vi "Extended Power Spectra 2D.vi"(8 "Error In":errorcluster, 9 "Waveforms In":waveform(dbl)[](array[waveform])) -> (0 "Error Out":errorcluster, 1 "Power Spectra":cluster{"f0":dbl, "df":dbl, "Magnitude":dbl[]}[](array[cluster]), 2 "Power Spectra 2":cluster{"f0":dbl, "df":dbl, "Magnitude":dbl[]}, 3 "Power Spectra 1":cluster{"f0":dbl, "df":dbl, "Magnitude":dbl[]})   [LabVIEW 2017]
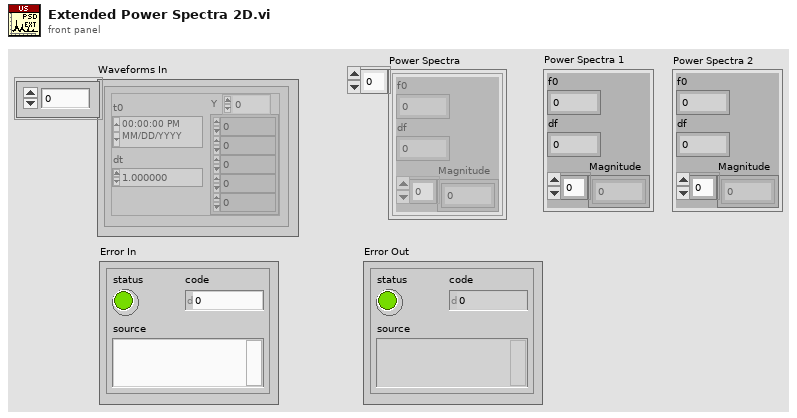
[diagram p1: front panel]
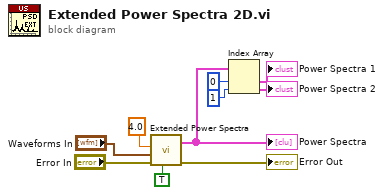
[diagram p0: block diagram]
diagram:
  n1 = call "Extended Power Spectra.vi"("Normalize?"=TRUE, "Error In"="Error In", "Waveforms In"="Waveforms In", "Upsampling pow. of 2"=4.0) -> ("Error Out"=→"Error Out":errorcluster, "Power Spectra"=w7:cluster{"f0":dbl, "df":dbl, "Magnitude":dbl[]}[])  [unwired: 6 in]
  "Power Spectra" <- w7
  n2 = Index Array(array=w7, index #1=0 ("disabled index (col)"), index #2=1 ("index (col)")) -> (element #1=→"Power Spectra 1":cluster{"f0":dbl, "df":dbl, "Magnitude":dbl[]}, element #2=→"Power Spectra 2":cluster{"f0":dbl, "df":dbl, "Magnitude":dbl[]})
